vi "align.vi"(6 "KickTarget":dbl[](array[numeric]), 8 "error in (no error)":errorcluster, 9 "Ball":refnum<class "Ball.lvclass">, 10 "Robot":refnum<class "Robot.lvclass">, 11 "KickToSkill in":refnum<class "KickToSkill.lvclass">) -> (0 "error out":errorcluster, 2 "Robot out":refnum<class "Robot.lvclass">, 3 "KickToSkill out":refnum<class "KickToSkill.lvclass">)   [LabVIEW 2023, in "KickToSkill.lvclass"]
uses:
  KickToSkill.lvclass
  Robot_class/Robot.lvclass
  Ball_class/Ball.lvclass
  C:/Users/ebert/Desktop/roboime/SSL_AI/Object_class/Object.lvclass
  Object_class/Object.lvclass/Object.ctl
  Robot_class/Robot.lvclass/Robot.ctl
  <vilib>/Analysis/baseanly.llb/Unit Vector (DBL).vi
  Object_class/Read position(x,y).vi
  Robot_class/Write dest_x.vi
  Robot_class/Write dest_y.vi
  Robot_class/Write dest_orientation.vi
  <vilib>/Analysis/NI_AALBase.lvlib
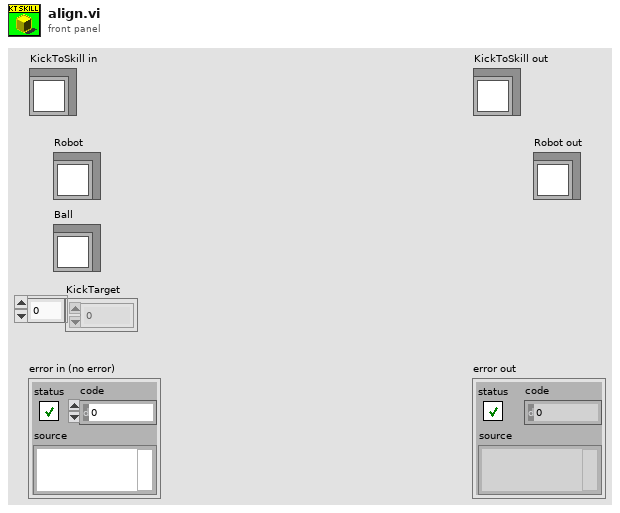
[diagram p1: front panel]
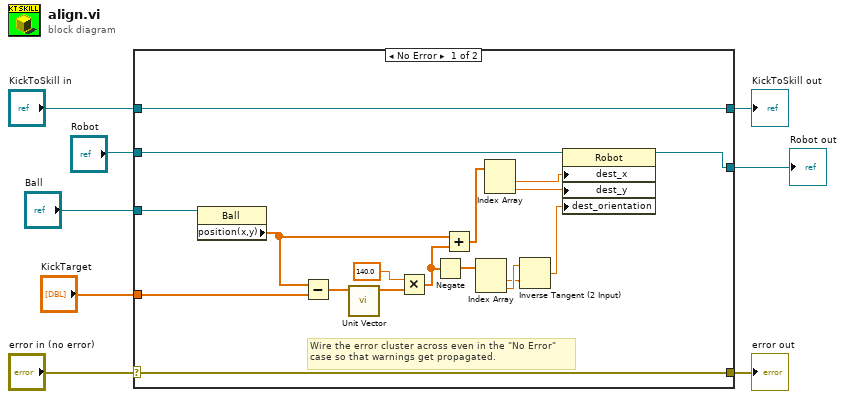
[diagram p0: block diagram]
diagram:
  n1 = case shown="No Error" "error in (no error)" {
    selector: "error in (no error)" -> [w25 w29]
    tunnel: [w25 w29] -> w7
    tunnel: [w26 w28] -> w5
    tunnel: "KickToSkill in" -> [w26 w28]
    tunnel: [w12 w27] -> w4
    tunnel: "Robot" -> [w11 w27]
    tunnel: "Ball" -> [w10 _]
    tunnel: "KickTarget" -> [w9 _]
    frame No Error {
      # "Wire the error cluster across even in the \"No Error\"\ncase so that warnings get propagated."
      n2 = property class="Ball"(reference=w10) -> ("position(x,y)"=w23:dbl[])  [unwired: 1 in, 2 out]
      n3 = Subtract(x=w23, y=w9) -> (x-y=w24:dbl[])
      n4 = call-poly <vilib>:"Unit Vector.vi"("Input Vector"=w24) -> ("Unit Vector"=w21:dbl[])  [unwired: 8 in, 2 out]
      n5 = Multiply(x=140.0, y=w21) -> (x*y=w14:dbl[])
      n6 = Negate(x=w14) -> (-x=w13:dbl[])
      n7 = Add(x=w23, y=w14) -> (x+y=w20:dbl[])
      n8 = Index Array(array=w13) -> (element #1=w16:dbl, element #2=w17:dbl)  [unwired: 2 in]
      n9 = Index Array(array=w20) -> (element #1=w19:dbl, element #2=w18:dbl)  [unwired: 2 in]
      n10 = Inverse Tangent (2 Input)(1:w16, 2:w17) -> (0:w15:dbl)
      n11 = property class="Robot"(reference=w11, "dest_x"=w19, "dest_y"=w18, "dest_orientation"=w15) -> (reference out=w12:refnum<class "Robot.lvclass">)  [unwired: 1 in, 1 out]
    }
    frame Error {
    }
  }
  "error out" <- w7
  "KickToSkill out" <- w5
  "Robot out" <- w4
